vi "Flatness_Load-Pairs.vi"(0 "Session In":refnum<visa-resource-name>="TCPIP0::169.254.70.100::inst0::INSTR", 1 "Timeout":u32=3000, 5 "error in":errorcluster {"code" format="%.0x"}, 7 "Freq":dbl=20.0, 9 "Freq Units":u16(ring) items=["Hz", "MHz", "GHz"], 11 "corr":dbl, 13 "corr unit":string(combo)="dB") -> (14 "Session Out":refnum<visa-resource-name>="TCPIP0::169.254.70.100::inst0::INSTR", 19 "error out":errorcluster {"code" format="%.0x"})   [LabVIEW 2018]
doc: "Launches the Instrument I/O Assistant, which you can use to communicate with message-based instruments and graphically parse the response. For example you can communicate with an instrument that uses a serial, Ethernet, or GPIB interface."
panel:
  # "Keysight MXG/EXG USER FLATNESS"
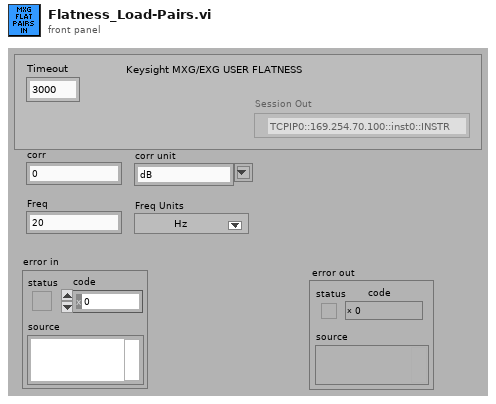
[diagram p1: front panel]
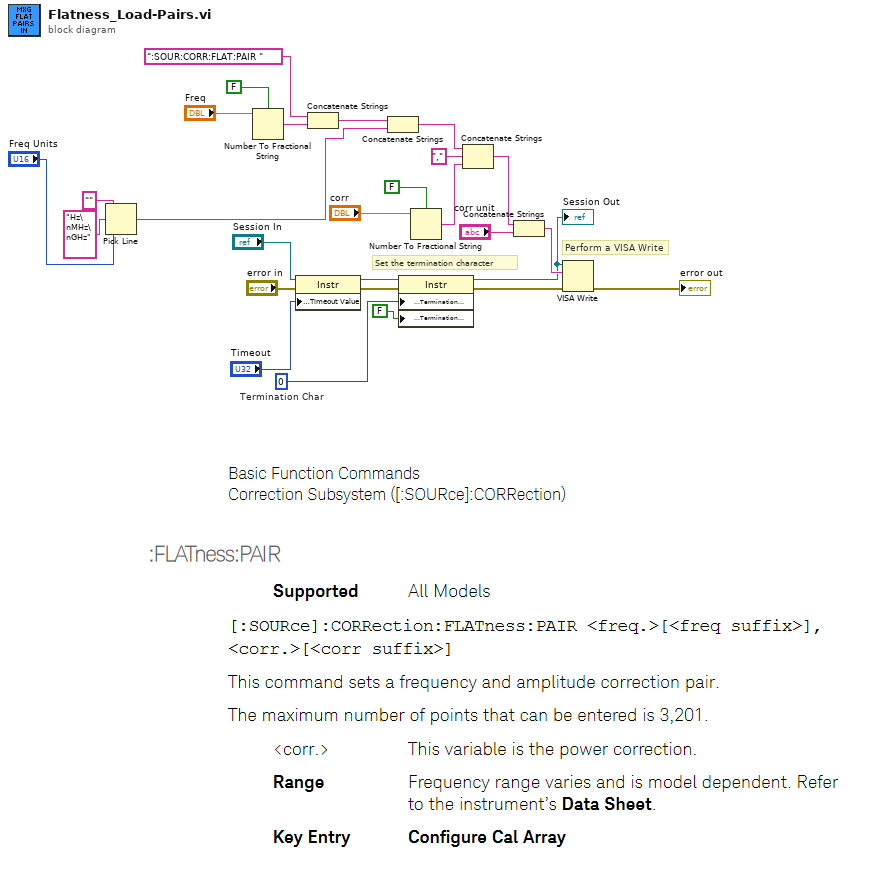
[diagram p0: block diagram]
diagram:
  w18 = u8 0  # Termination Char
  # "Perform a VISA Write"
  # "Set the termination character"
  n1 = Pick Line(string ("")="", multi-line string="Hz\nMHz\nGHz", line index="Freq Units") -> (output string=w3:string)
  n2 = Number To Fractional String(use system decimal point (T)=FALSE, number="Freq") -> (F-format string=w15:string)  [unwired: 2 in]
  n3 = property class="Instr"(reference="Session In", error in="error in", "General Settings:Timeout Value"="Timeout") -> (reference out=w17:refnum<visa-resource-name>, error out=w20:errorcluster)
  n4 = Concatenate Strings(":SOUR:CORR:FLAT:PAIR " ("staticText"), w15) -> (w13:string)
  n5 = Concatenate Strings(w13, w3) -> (w11:string)
  n6 = property class="Instr"(reference=w17, error in=w20, "Message Based Settings:Termination Character"=w18, "Message Based Settings:Termination Character Enable"=FALSE ("enable")) -> (reference out=w5:refnum<visa-resource-name>, error out=w19:errorcluster)
  "Session Out" <- w5
  n7 = Number To Fractional String(use system decimal point (T)=FALSE, number="corr") -> (F-format string=w12:string)  [unwired: 2 in]
  n8 = Concatenate Strings(w11, "," ("staticText"), w12) -> (w8:string)
  n9 = Concatenate Strings(w8, "corr unit") -> (w6:string)
  n10 = VISA Write(VISA resource name=w5, write buffer=w6, error in (no error)=w19) -> (error out=→"error out":errorcluster)  [unwired: 2 out]
